vi "final Vi_3.vi"() -> ()   [LabVIEW 2018]
uses:
  <vilib>/Utility/file.llb/Read Delimited Spreadsheet (string).vi
  <vilib>/Utility/file.llb/Read Delimited Spreadsheet (DBL).vi
  <vilib>/Analysis/3filter.llb/Equi-Ripple BandPass (DBL).vi
  <vilib>/Analysis/NI_AALBase.lvlib
  <vilib>/Analysis/NI_AAL_SigProc.lvlib
panel:
  out "yeee":dbl[](array[numeric])
  out "我們計算的RR":cluster{i32[], dbl[]}(graph)
  out "Array":dbl[](array[numeric])
  in  "threshold":dbl=10000.0 format="%0.2f"
  out "Locations":dbl[](array[numeric])
  in  "filter higher  stop freq":dbl(slide)=0.4094594594594595 scale=0.4..0.5
  out "平均心跳/分鐘":dbl
  out "?":bool
  out "RMSSD(ms)":dbl
  out "HR":cluster{i32[], dbl[]}[](graph)
  out "Mean R-R interval":dbl
  out "RR":cluster{dbl[], dbl[]}(graph)
  in  "filter lower stop freq":dbl(slide)=0.032972972972972976 scale=0.0..0.1
  out "Band filter":cluster{dbl[], "Filtered X":dbl[]}[](graph)
  out "Origin ECG":cluster{dbl[], i32[]}(graph)
  # "RMSSD越大，\n表示副交感神經作用越強"
  # "一般正常心跳約為50~100下/分鐘"
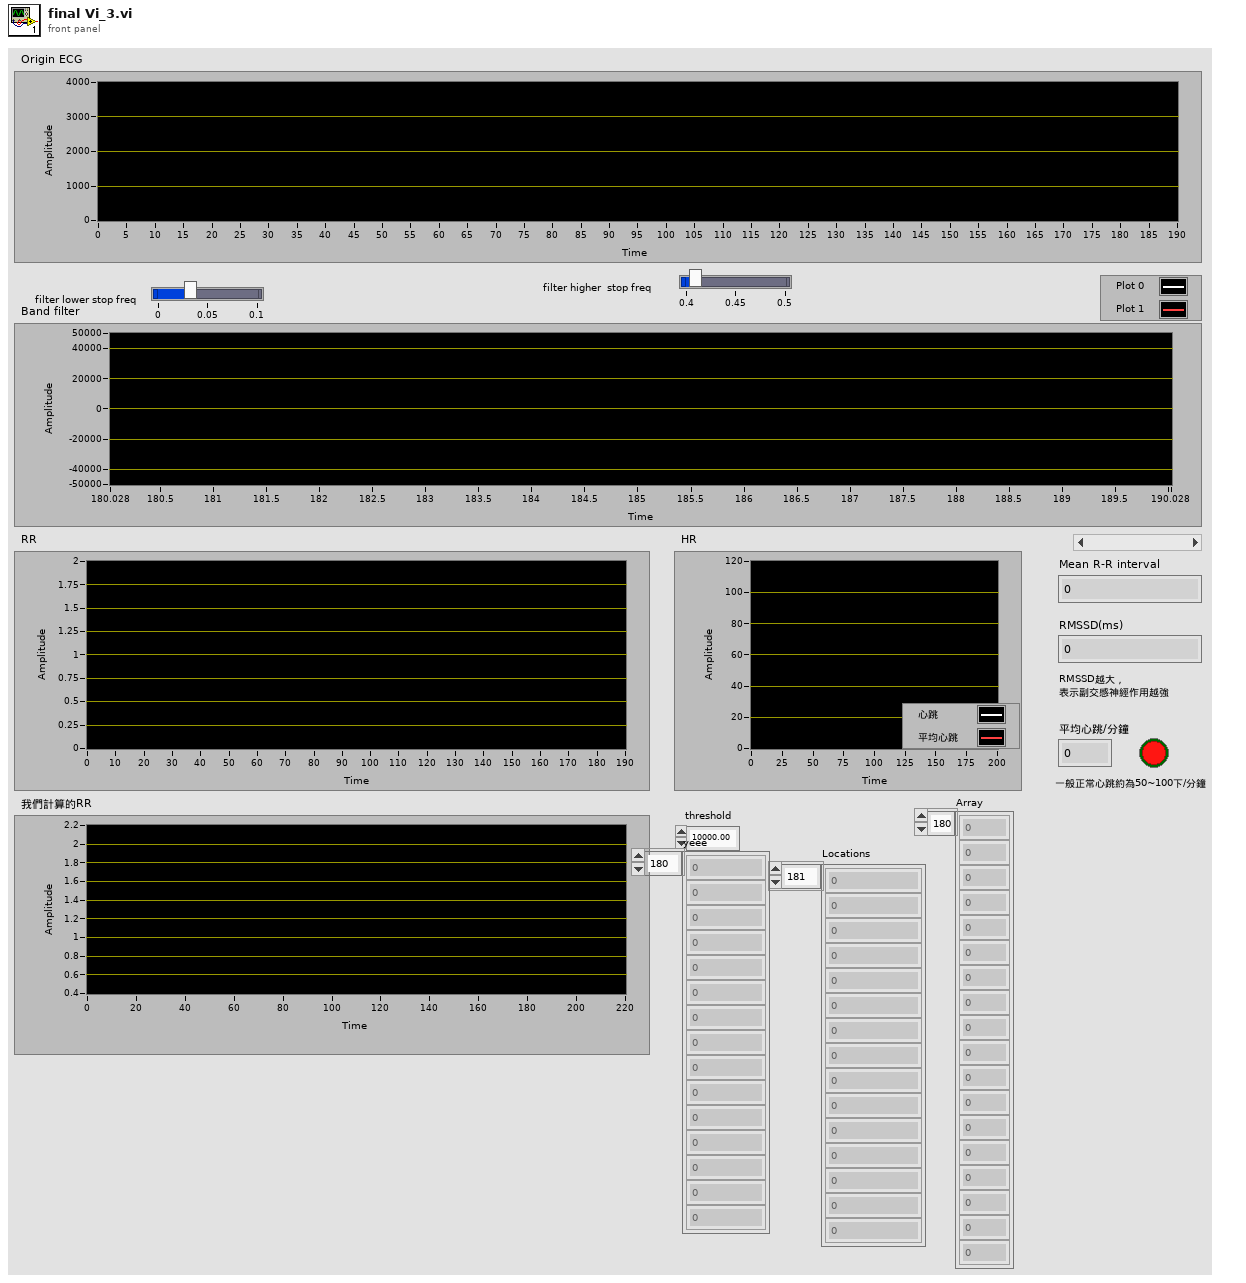
[diagram p1: front panel]
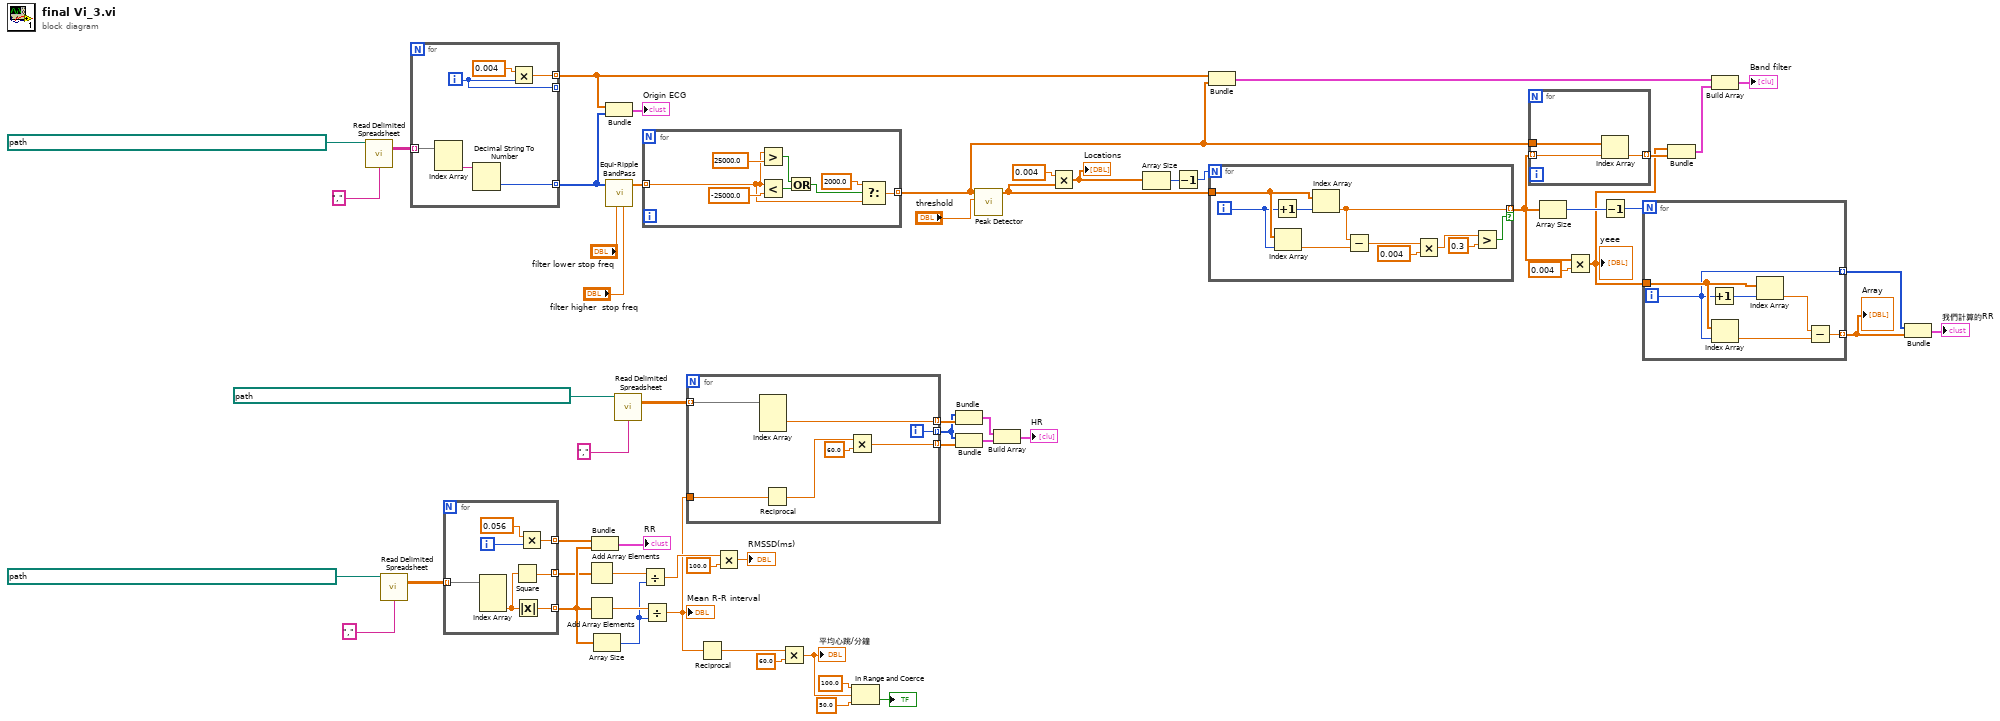
[diagram p0: block diagram]
diagram:
  n1 = call-poly <vilib>:"Read Delimited Spreadsheet.vi"("file path (dialog if empty)"=path "D:/Documents/生醫儀表/data/2019_05_25__16_08_04_ECG.csv", "delimiter (\\t)"="," ("delimiter (\\t)")) -> ("all rows"=w56:string[][])  [unwired: 8 in, 5 out]
  n2 = call-poly <vilib>:"Read Delimited Spreadsheet.vi"("file path (dialog if empty)"=path "D:/Documents/生醫儀表/data/2019_05_25__16_08_04_BR_RR.csv", "delimiter (\\t)"="," ("delimiter (\\t)")) -> ("all rows"=w53:dbl[][])  [unwired: 8 in, 5 out]
  n3 = for {
    tunnel: w56 -> [w63] mode=indexing
    tunnel: [w62] -> w20 mode=indexing
    tunnel: [w60] -> w14 mode=indexing
    tunnel: [w58] -> _ mode=indexing
    i -> [w58]
    n4 = Index Array(array=w63) -> (element #2=w59:string)  [unwired: 2 in, 1 out]
    n5 = Decimal String To Number(string=w59) -> (number=w62:i32)  [unwired: 2 in, 1 out]
    n6 = Multiply(x=0.004 ("y"), y=w58) -> (x*y=w60:dbl)
  }
  n7 = for {
    tunnel: w53 -> [w70] mode=indexing
    tunnel: [w67] -> w51 mode=indexing
    tunnel: [w66] -> w47 mode=indexing
    tunnel: [w64] -> w37 mode=indexing
    i -> [w69]
    n8 = Index Array(array=w70) -> (element #3=w65:dbl)  [unwired: 3 in, 2 out]
    n9 = Square(x=w65) -> (x^2=w64:dbl)
    n10 = Absolute Value(x=w65) -> (abs(x)=w66:dbl)
    n11 = Multiply(x=0.056 ("y"), y=w69) -> (x*y=w67:dbl)
  }
  n12 = Add Array Elements(numeric array=w37) -> (sum=w36:dbl)
  n13 = Add Array Elements(numeric array=w47) -> (sum=w48:dbl)
  n14 = Bundle(w51, w47) -> (→"RR":cluster{dbl[], dbl[]})  [unwired: 1 in]
  n15 = Array Size(array=w47) -> (size(s)=w35:i32)
  n16 = Bundle(w14, w20) -> (→"Origin ECG":cluster{dbl[], i32[]})  [unwired: 1 in]
  n17 = call-poly <vilib>:"Equi-Ripple BandPass.vi"("X"=w20, "lower stop freq"="filter lower stop freq", "higher stop freq"="filter higher  stop freq") -> ("Filtered X"=w8:dbl[])  [unwired: 5 in, 1 out]
  n18 = call-poly <vilib>:"Read Delimited Spreadsheet.vi"("file path (dialog if empty)"=path "D:/Documents/生醫儀表/data/2019_05_25__16_08_04_General.csv", "delimiter (\\t)"="," ("delimiter (\\t)")) -> ("all rows"=w44:dbl[][])  [unwired: 8 in, 5 out]
  n19 = Divide(x=w36, y=w35) -> (x/y=w34:dbl)
  n20 = for {
    tunnel: w8 -> [w72] mode=indexing
    tunnel: [w71] -> w7 mode=indexing
    n21 = Greater?(x=w72, y=25000.0) -> (0:w76:bool)
    n22 = Less?(x=w72, y=-25000.0) -> (x < y?=w75:bool)
    n23 = Or(x=w76, y=w75) -> (x .or. y?=w74:bool)
    n24 = Select(t=2000.0, s=w74, f=w72) -> (s? t:f=w71:dbl)
  }
  n25 = Divide(x=w48, y=w35) -> (x/y=w29:dbl)
  "Mean R-R interval" <- w29
  n26 = for {
    tunnel: w44 -> [w85] mode=indexing
    tunnel: [w84] -> w43 mode=indexing
    tunnel: [w83] -> w42 mode=indexing
    tunnel: w29 -> [w82]
    tunnel: [w79] -> w38 mode=indexing
    i -> [w83]
    n27 = Index Array(array=w85) -> (element #2=w84:dbl)  [unwired: 3 in, 2 out]
    n28 = Reciprocal(x=w82) -> (1/x=w81:dbl)
    n29 = Multiply(x=w81, y=60.0) -> (x*y=w79:dbl)
  }
  n30 = Reciprocal(x=w29) -> (1/x=w31:dbl)
  n31 = Multiply(x=w34, y=100.0) -> (x*y=→"RMSSD(ms)":dbl)
  n32 = Multiply(x=w31, y=60.0) -> (x*y=w28:dbl)
  "平均心跳/分鐘" <- w28
  n33 = In Range and Coerce(upper limit=100.0, x=w28, lower limit=50.0) -> (In Range?=→"?":bool)  [unwired: 1 out]
  n34 = Bundle(w42, w43) -> (w41:cluster{i32[], dbl[]})  [unwired: 1 in]
  n35 = Bundle(w42, w38) -> (w39:cluster{i32[], dbl[]})  [unwired: 1 in]
  n36 = call <vilib>:"Peak Detector.vi"("threshold"="threshold", "X"=w7) -> ("Locations"=w1:dbl[])  [unwired: 5 in, 4 out]
  n37 = Build Array(w41, w39) -> (→"HR":cluster{i32[], dbl[]}[])
  n38 = Multiply(x=0.004 ("y"), y=w1) -> (x*y=w12:dbl[])
  "Locations" <- w12
  n39 = Array Size(array=w12) -> (size(s)=w13:i32)
  n40 = Decrement(x=w13) -> (x-1=w4:i32)
  n41 = Bundle(w14, w7) -> (w18:cluster{dbl[], dbl[]})  [unwired: 1 in]
  n42 = for {
    N: w4 -> [_]
    tunnel: w1 -> [w95]
    tunnel: [w86] -> w3 mode=indexing if=w88
    i -> [w94]
    n43 = Increment(x=w94) -> (x+1=w93:i32)
    n44 = Index Array(array=w95, index=w94) -> (element=w87:dbl)
    n45 = Index Array(array=w95, index=w93) -> (element=w86:dbl)
    n46 = Subtract(x=w86, y=w87) -> (x-y=w91:dbl)
    n47 = Multiply(x=w91, y=0.004) -> (x*y=w90:dbl)
    n48 = Greater?(x=w90, y=0.3) -> (0:w88:bool)
  }
  n49 = for {
    tunnel: w3 -> [w97] mode=indexing
    tunnel: w7 -> [w98]
    tunnel: [w96] -> w16 mode=indexing
    n50 = Index Array(array=w98, index=w97) -> (element=w96:dbl)
  }
  n51 = Array Size(array=w3) -> (size(s)=w10:i32)
  n52 = Multiply(x=w3, y=0.004) -> (x*y=w2:dbl[])
  "yeee" <- w2
  n53 = Decrement(x=w10) -> (x-1=w9:i32)
  n54 = for {
    N: w9 -> [_]
    tunnel: w2 -> [w104]
    tunnel: [w100] -> w5 mode=indexing
    tunnel: [w99] -> w21 mode=indexing
    i -> [w99]
    n55 = Increment(x=w99) -> (x+1=w103:i32)
    n56 = Index Array(array=w104, index=w99) -> (element=w101:dbl)
    n57 = Index Array(array=w104, index=w103) -> (element=w102:dbl)
    n58 = Subtract(x=w102, y=w101) -> (x-y=w100:dbl)
  }
  "Array" <- w5
  n59 = Bundle(w2, w16) -> (w15:cluster{dbl[], dbl[]})  [unwired: 1 in]
  n60 = Build Array(w18, w15) -> (→"Band filter":cluster{dbl[], dbl[]}[])
  n61 = Bundle(w21, w5) -> (→"我們計算的RR":cluster{i32[], dbl[]})  [unwired: 1 in]
